vi "Populate Ctl by Query.vi"(8 "error in (no error)":errorcluster, 10 "SQL Query (use builtin)":string, 11 "FK Ring in":refnum<class "FK Ring.lvclass">) -> (0 "error out":errorcluster, 3 "FK Ring out":refnum<class "FK Ring.lvclass">)   [LabVIEW 2020, in "FK Ring.lvclass"]
uses:
  FK Ring.lvclass
  C:/Users/User/Desktop/Raman Program/Database OOP/source/Field/Field.lvclass
  C:/Users/User/Desktop/Raman Program/Database OOP/source/Ring Field/Ring Field.lvclass
  Field/Field.lvclass/Field.ctl
  FK Ring.lvclass/FK Ring.ctl
  Ring Field/Set Ring Strings and Values by Table.vi
  Database/Database.lvclass
  Field/Field.lvclass
  C:/Users/User/Desktop/Raman Program/Database OOP/source/FK Ring/FK Ring.lvclass
  Ring Field/Ring Field.lvclass
panel:
  # "Use this method to populate a field using a query.\nIf no query is supplied, then use dynamic dispatch to build\nan appropriate query from child member data.\nIf the field has nothing to populate, do not implement method."
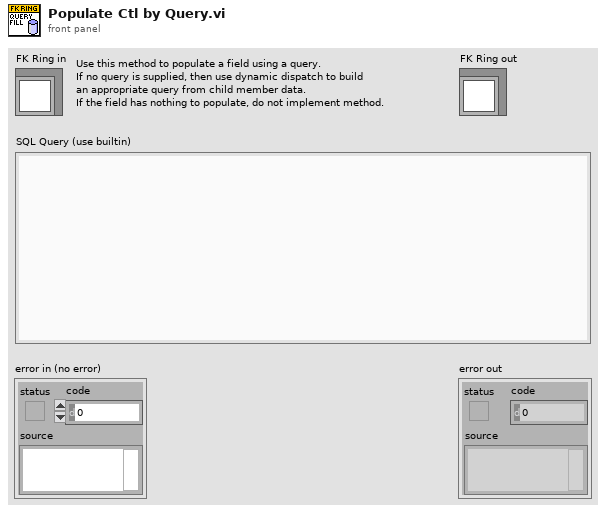
[diagram p1: front panel]
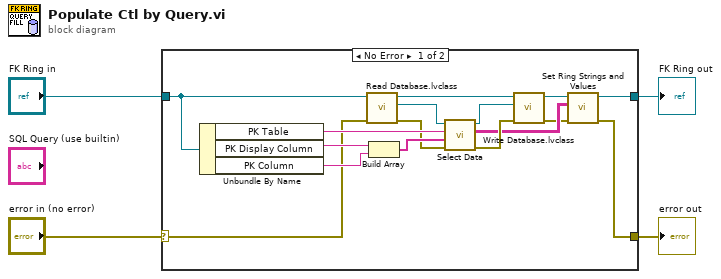
[diagram p0: block diagram]
diagram:
  n1 = case shown="No Error" "error in (no error)" {
    selector: "error in (no error)" -> [w10 w22]
    tunnel: [w5 w22] -> w3
    tunnel: "FK Ring in" -> [w20 w21]
    tunnel: [w8 w21] -> w1
    frame No Error {
      n2 = Unbundle By Name(w20) -> ("PK Table"=w13:string, "PK Display Column"=w16:string, "PK Column"=w15:string)
      n3 = call "Read Database.lvclass.vi"("error in (no error)"=w10, "Field in"=w20) -> ("error out"=w12:errorcluster, "Database.lvclass"=w18:refnum<class "Database.lvclass">, "Field out"=w19:refnum<class "FK Ring.lvclass">)  [unwired: 7 in]
      n4 = Build Array(w16, w15) -> (w14:string[])
      n5 = call-dynamic "Select Data.vi"("error in (no error)"=w12, "Columns"=w14, "Table"=w13, "Database in"=w18) -> ("error out"=w11:errorcluster, "Data"=w7:string[][], "Database out"=w17:refnum<class "Database.lvclass">)  [unwired: 5 in]
      n6 = call "Write Database.lvclass.vi"("error in (no error)"=w11, "Database.lvclass"=w17, "Field in"=w19) -> ("error out"=w6:errorcluster, "Field out"=w9:refnum<class "FK Ring.lvclass">)  [unwired: 7 in]
      n7 = call-poly "Set Ring Strings and Values.vi"("error in (no error)"=w6, "String and Values"=w7, "Ring Field in"=w9) -> ("error out"=w5:errorcluster, "Ring Field out"=w8:refnum<class "FK Ring.lvclass">)  [unwired: 7 in]
    }
    frame Error {
    }
  }
  "error out" <- w3
  "FK Ring out" <- w1
